vi "Ultrasonic Info.vi"   [LabVIEW 2016]
uses:
  <vilib>/Rock Robotics/WPI/Ultrasonic/WPI_SonarSRF04DigitalOpen.vi
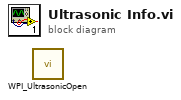
[diagram p0: block diagram]
diagram:
  n1 = call-poly <vilib>:"WPI_UltrasonicOpen.vi"() -> ()  [unwired: 10 in, 2 out]
